vi "getConfigurationType.vi"(0 "niDAQmxAO in":refnum<class "niDAQmxAO.lvclass">, 1 "error in (no error)":errorcluster) -> (2 "niDAQmxAO out":refnum<class "niDAQmxAO.lvclass">, 3 "Configuration Type":string, 4 "error out":errorcluster)   [LabVIEW 2011, in "Hardware.lvlib" / "Channels.lvlib" / "niDAQmxAO.lvclass"]
uses:
  niDAQmxAO.lvclass
  niDAQmxAO.lvclass/niDAQmxAO.ctl
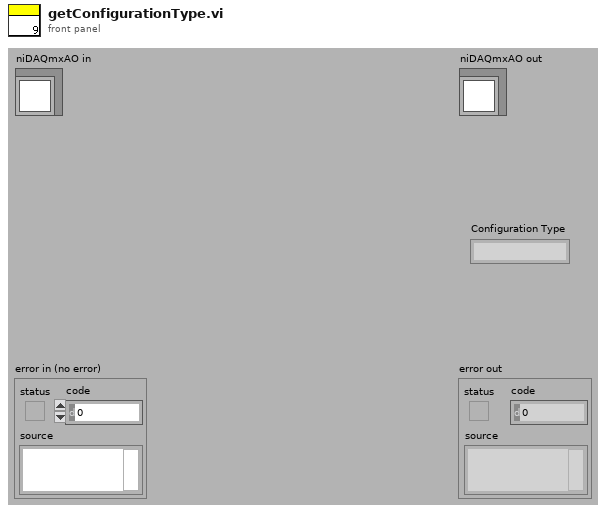
[diagram p1: front panel]
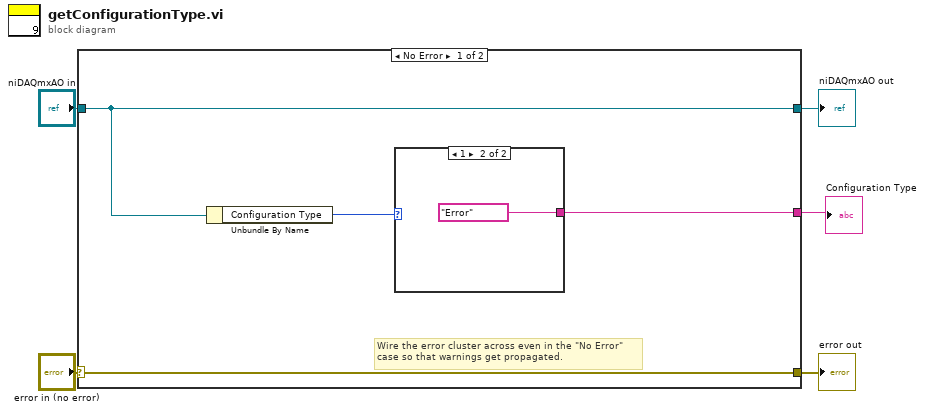
[diagram p0: block diagram]
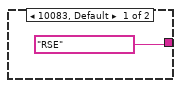
[diagram p2: hidden frame]
diagram:
  n1 = case shown="No Error" "error in (no error)" {
    selector: "error in (no error)" -> [w9 w13]
    tunnel: [w9 w13] -> w4
    tunnel: [w8 w12] -> w2
    tunnel: "niDAQmxAO in" -> [w8 w12]
    tunnel: [w6 _] -> w1
    frame No Error {
      # "Wire the error cluster across even in the \"No Error\"\ncase so that warnings get propagated."
      n2 = Unbundle By Name(w8) -> ("Configuration Type"=w7:u16)
      n3 = case shown="1" w7 {
        tunnel: ["RSE" "Error"] -> w6
        frame 10083, Default {
        }
        frame 1 {
        }
      }
    }
    frame Error {
    }
  }
  "error out" <- w4
  "niDAQmxAO out" <- w2
  "Configuration Type" <- w1
